vi "Email_Text_Files.vi"(0 "Filenames":path[](array[path]), 1 "message":string, 2 "subject ([No Subject])":string="[No Subject]") -> ()   [LabVIEW 2010]
uses:
  Email_transfer_global.vi
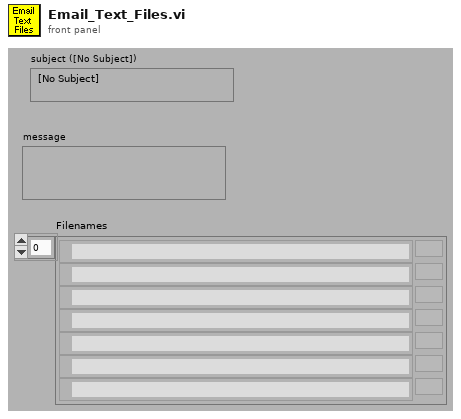
[diagram p1: front panel]
types:
  T1 = cluster{"path":path, "data":string, "binary":bool, "MIME content-type \n(application/octet-stream)":string}[]
  T2 = cluster{"path":path, "data":string, "binary":bool, "MIME content-type \n(application/octet-stream)":string}
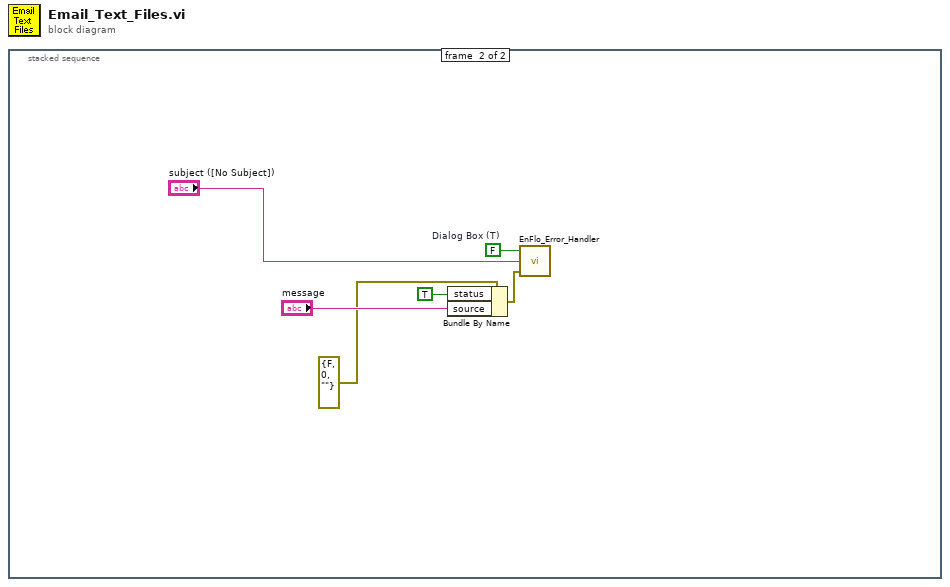
[diagram p0: block diagram]
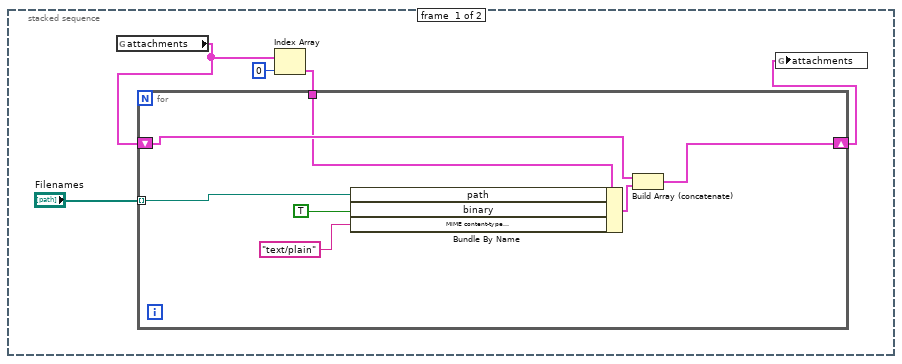
[diagram p2: hidden frame]
diagram:
  n1 = stacked-sequence {
    frame #0 {
      n2 = global read "Email_transfer_global.vi" "attachments"() -> (w4:T1)
      n3 = Index Array(array=w4, index=0) -> (element=w3:T2)
      n4 = for {
        shift-right: [w7] -> w2
        shift-left: w4 -> [w9]
        tunnel: w3 -> [w8]
        tunnel: "Filenames" -> [w6] mode=indexing
        n5 = Bundle By Name(cluster=w8, "path"=w6, "binary"=TRUE, "MIME content-type \n(application/octet-stream)"="text/plain" ("MIME content-type \n(application/octet-stream)")) -> (w10:T2)
        n6 = Build Array (concatenate)(w9, w10) -> (w7:T1)
      }
      n7 = global write "Email_transfer_global.vi" "attachments"(w2) -> ()
    }
    frame #1 {
      w18 = FALSE  # Dialog Box (T)
      n8 = Bundle By Name(cluster=errorcluster {"status"=FALSE, "code"=0, "source"=""} ("error in (no error)"), "status"=TRUE, "source"="message") -> (w15:errorcluster)
      n9 = call "EnFlo_Error_Handler.vi"("error in (no error)"=w15, "Error Type"="subject ([No Subject])", "Dialog Box (T)"=w18) -> ()  [unwired: 3 out]
    }
  }
